vi "ResumeConfig.vi"(8 "error in (no error)":errorcluster caption="错误输入（无错误）", 9 "CANInd":u32, 10 "DeciceInd":u32, 11 "DeviceType":u32) -> (0 "error out":errorcluster caption="错误输出", 3 "Success":bool)   [LabVIEW 2011]
uses:
  data/ControlCAN.dll
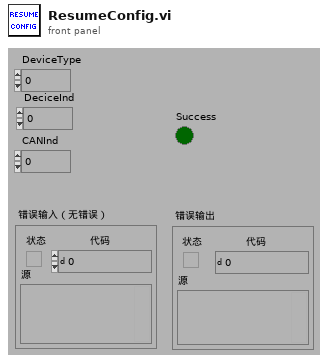
[diagram p1: front panel]
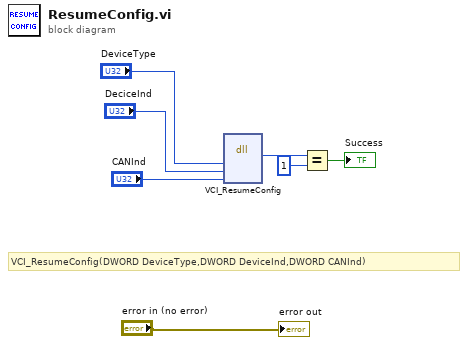
[diagram p0: block diagram]
diagram:
  # "VCI_ResumeConfig(DWORD DeviceType,DWORD DeviceInd,DWORD CANInd)"
  n1 = dll-call lib="PTH1Nabs D\t董海成\t上位机2.进行中USB-CAN TooldataControlCAN.dll" fn="VCI_ResumeConfig"("DeviceType"="DeviceType", "DeciceInd"="DeciceInd", "CANInd"="CANInd") -> ("返回类型"=w4:u32)  [unwired: 6 in, 2 out]
  n2 = Equal?(x=w4, y=u32 1) -> (x = y?=→"Success":bool)
  "error out" <- "error in (no error)"
